vi "EZ Current.vi"(6 "DC/AC (F:DC)":bool, 7 "Scan List (empty)":string, 8 "error in (no error)":errorcluster, 9 "Range (3:Auto)":T2(ring)=enum."Auto", 10 "Resolution (3:Least)":T1(ring)=enum."Least", 11 "VISA Resource Name":refnum<visa-resource-name>) -> (0 "error out":errorcluster, 2 "Output Array":dbl[](array[numeric]) format="%.2f", 3 "VISA Resource Name Out":refnum<visa-resource-name>)   [LabVIEW 2017, in "Agilent 34970.lvlib"]
doc: "This VI lets you take simple current measurements. This VI is only valid for channels 21 and 22 on the 34901 A module."
uses:
  <instrlib>/Agilent 34970/Agilent 34970.lvlib
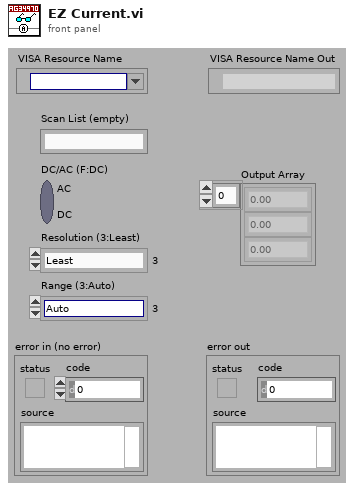
[diagram p1: front panel]
types:
  T1 = enum16{"4 1/2", "5 1/2", "6 1/2", "Least", "Highest", "Default"}
  T2 = enum16{"10 mA", "100 mA", "1 A", "Auto", "Minimum", "Maximum"}
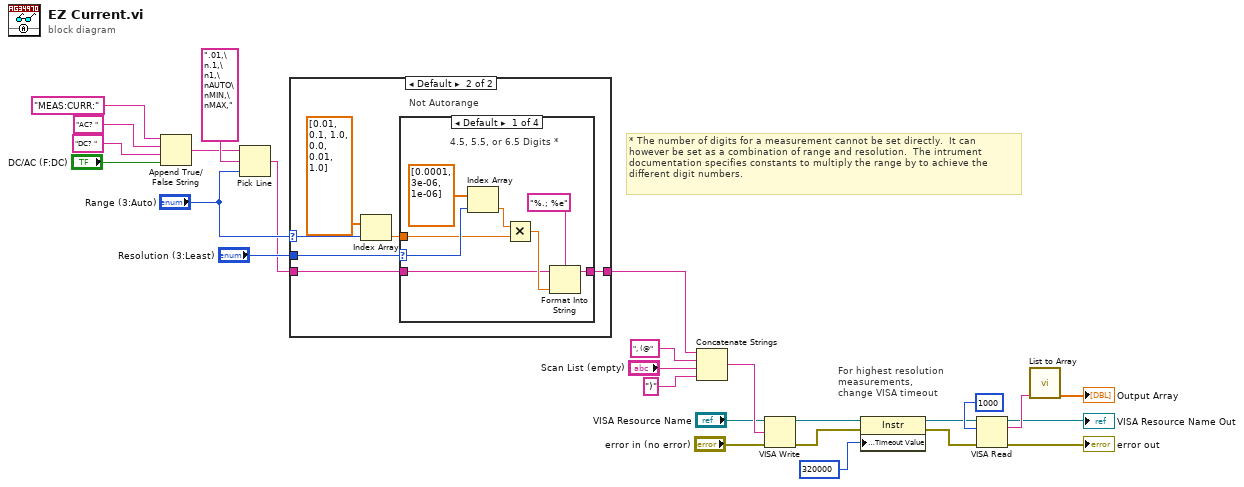
[diagram p0: block diagram]
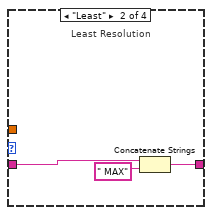
[diagram p3: hidden frame]
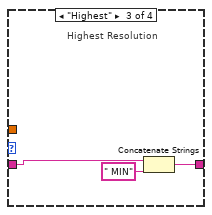
[diagram p4: hidden frame]
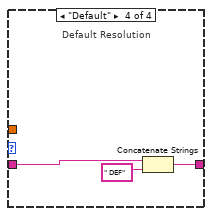
[diagram p5: hidden frame]
diagram:
  # "* The number of digits for a measurement cannot be set directly.  It can\nhowever be set as a combination of range and resolution.  The intrument\ndocumentation specifies constants to multiply the range by to achieve the\ndifferent digit numbers."
  # "For highest resolution\nmeasurements, \nchange VISA timeout"
  n1 = Append True/False String(1:"DC/AC (F:DC)", 2:"DC? ", 3:"AC? ", 4:"MEAS:CURR:") -> (0:w13:string)
  n2 = Pick Line(string ("")=w13, multi-line string=".01,\n.1,\n1,\nAUTO\nMIN,\nMAX,", line index="Range (3:Auto)") -> (output string=w2:string)
  n3 = case shown="Default" "Range (3:Auto)" {
    selector: "Range (3:Auto)" -> [_ w31]
    tunnel: "Resolution (3:Least)" -> [_ w30]
    tunnel: w2 -> [w27 w29]
    tunnel: [w27 w28] -> w1
    frame "Auto" {
      # "Autorange"
    }
    frame Default {
      # "Not Autorange"
      n4 = Index Array(array=dbl[] [0.01, 0.1, 1.0, 0.0, 0.01, 1.0], index=w31) -> (element=w33:dbl)
      n5 = case shown="Default" w30 {
        selector: w30 -> [w40 _ _ _]
        tunnel: [w35 w44 w47 w49] -> w28
        tunnel: w33 -> [w39 _ _ _]
        tunnel: w29 -> [w34 w42 w45 w48]
        frame Default {
          # "4.5, 5.5, or 6.5 Digits *"
          n6 = Index Array(array=dbl[] [0.0001, 3e-06, 1e-06], index=w40) -> (element=w38:dbl)
          n7 = Multiply(x=w38, y=w39) -> (x*y=w37:dbl)
          n8 = Format Into String(format string="%.; %e", initial string=w34, w37) -> (resulting string=w35:string)  [unwired: 1 in, 1 out]
        }
        frame "Least" {
          # "Least Resolution"
          n9 = Concatenate Strings(w42, " MAX" ("string")) -> (w44:string)
        }
        frame "Highest" {
          # "Highest Resolution"
          n10 = Concatenate Strings(w45, " MIN" ("string")) -> (w47:string)
        }
        frame "Default" {
          # "Default Resolution"
          n11 = Concatenate Strings(w48, " DEF" ("string")) -> (w49:string)
        }
      }
    }
  }
  n12 = Concatenate Strings(w1, ", (@", "Scan List (empty)", ")") -> (w19:string)
  n13 = VISA Write(VISA resource name="VISA Resource Name", write buffer=w19, error in (no error)="error in (no error)") -> (VISA resource name out=w23:refnum<visa-resource-name>, error out=w22:errorcluster)  [unwired: 1 out]
  n14 = property class="Instr"(reference=w23, error in=w22, "General Settings:Timeout Value"=u32 320000 ("Tmo Value")) -> (reference out=w20:refnum<visa-resource-name>, error out=w21:errorcluster)
  n15 = VISA Read(VISA resource name=w20, byte count=u32 1000 ("byte count (0)"), error in (no error)=w21) -> (VISA resource name out=→"VISA Resource Name Out":refnum<visa-resource-name>, read buffer=w12:string, error out=→"error out":errorcluster)  [unwired: 1 out]
  n16 = call <instrlib>:"List to Array.vi"("List (empty)"=w12) -> ("Output Number Array"=→"Output Array":dbl[])  [unwired: 9 in, 1 out]
